vi "沿线段检测边沿点2.vi"(6 "开启线段Overlay":bool, 7 "Edge Options":T3={"Edge Polarity"=0, "Kernel Size"=5, "Width"=11, "Minimum Edge Strength"=10.0, "Interpolation Type"=enum."Bilinear Fixed", "Data Processing Method"=enum."Average"} {"Edge Polarity" items=["All Edges", "Rising Edges", "Falling Edges"]; "Minimum Edge Strength" format="%.2f"; "Width" step=2; "Kernel Size" step=2}, 8 "error in (no error)":errorcluster, 9 "终点":cluster{"X":sgl, "Y":sgl}, 10 "起点":cluster{"X":sgl, "Y":sgl}, 11 "Image":T1) -> (0 "error out":errorcluster, 2 "Edge Information":T2[](array[typedef]) {"Distance (Real-World)" format="%.2f"; "Location (Real-World)"."Y" format="%.2g"; "Location (Real-World)"."X" format="%.2f"; "Noise" format="%.2f"; "Location (Pixel)"."Y" format="%.2g"; "Location (Pixel)"."X" format="%.2f"; "Strength" format="%.2f"; "Distance (Pixel)" format="%.2f"}, 3 "Image Out":T1)   [LabVIEW 2015]
uses:
  <vilib>/vision/Measure.llb/Edge Options.ctl
  <vilib>/vision/Measure.llb/Edge Polarity.ctl
  <vilib>/vision/Measure.llb/Edge New.ctl
  <vilib>/vision/Image Controls.llb/IMAQ Image.ctl
  <vilib>/vision/NI_Vision_Development_Module.lvlib
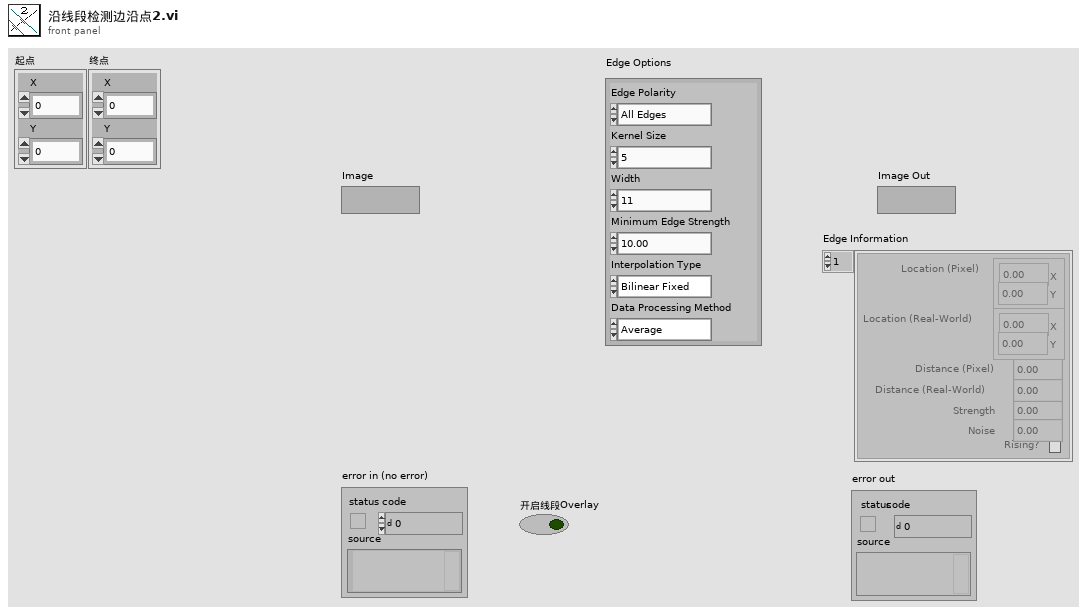
[diagram p1: front panel]
types:
  T1 = typedef "IMAQ Image.ctl" = refnum<image>
  T2 = typedef "Edge New.ctl" = cluster{"Location (Pixel)":cluster{"X":sgl, "Y":sgl}, "Location (Real-World)":cluster{"X":sgl, "Y":sgl}, "Distance (Pixel)":dbl, "Distance (Real-World)":dbl, "Strength":dbl, "Noise":dbl, "Rising?":bool}
  T3 = typedef "Edge Options.ctl" = cluster{"Edge Polarity":T4, "Kernel Size":u32, "Width":u32, "Minimum Edge Strength":sgl, "Interpolation Type":enum32{"Zero Order", "Bilinear", "Quadratic", "Cubic", "Bilinear Fixed"}, "Data Processing Method":enum32{"Average", "Median"}}
  T4 = typedef "Edge Polarity.ctl" = u32
  T5 = typedef "IMAQ Line" = cluster{"Start X":i32, "Start Y":i32, "End X":i32, "End Y":i32}
  T6 = typedef "ROI Descriptor" = cluster{"Global Rectangle":i32[], "Contours":cluster{"ID":enum32{"External", "Internal"}, "Type":u32, "Coordinates":i32[]}[]}
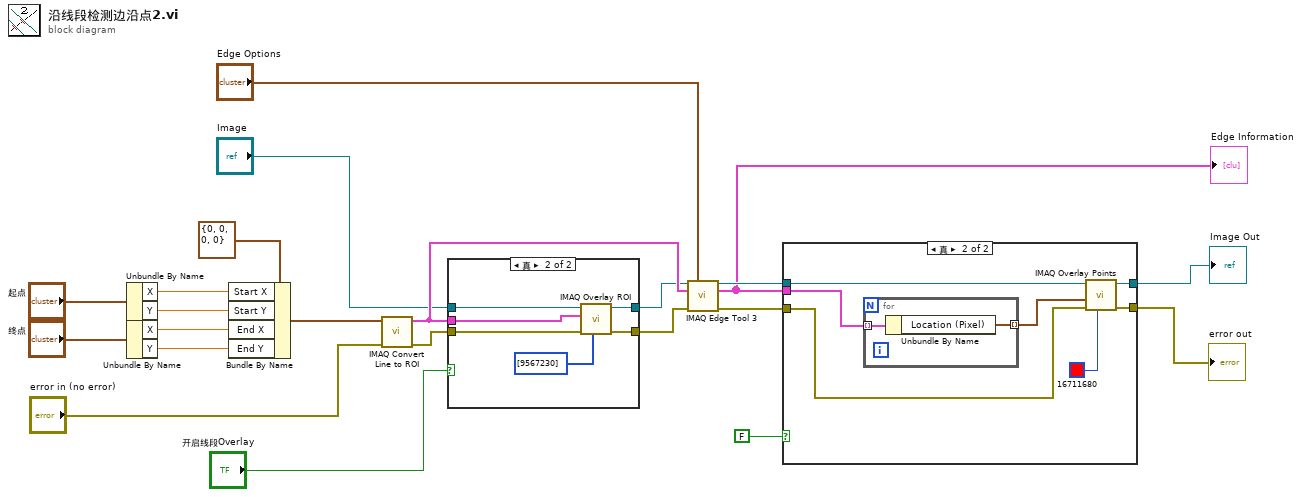
[diagram p0: block diagram]
diagram:
  n1 = Unbundle By Name("起点") -> ("X"=w6:sgl, "Y"=w5:sgl)
  n2 = Unbundle By Name("终点") -> ("X"=w3:sgl, "Y"=w2:sgl)
  n3 = Bundle By Name(cluster=T5 {"Start X"=0, "Start Y"=0, "End X"=0, "End Y"=0} ("Line"), "Start X"=w6, "Start Y"=w5, "End X"=w3, "End Y"=w2) -> (w8:T5)
  n4 = call "IMAQ Convert Line to ROI"("error in (no error)"="error in (no error)", "Line"=w8) -> ("error out"=w20:errorcluster, "ROI Descriptor"=w22:T6)  [unwired: 7 in]
  n5 = case shown="真" "开启线段Overlay" {
    tunnel: w22 -> [_ w29]
    tunnel: [w23 w28] -> w21
    tunnel: w20 -> [w24 w27]
    tunnel: [w24 w26] -> w19
    tunnel: "Image" -> [w23 w25]
    frame False {
    }
    frame True {
      n6 = call "IMAQ Overlay ROI"("Colors (Green)"=u32[] [9567230], "error in (no error)"=w27, "ROI Descriptor"=w29, "Image"=w25) -> ("error out"=w26:errorcluster, "Image Out"=w28:T1)  [unwired: 6 in]
    }
  }
  n7 = call "IMAQ Edge Tool 3"("Image"=w21, "Edge Options"="Edge Options", "ROI Descriptor"=w22, "error in (no error)"=w19) -> ("Image (duplicate)"=w17:T1, "Edge Information"=w11:T2[], "error out"=w14:errorcluster)  [unwired: 7 in, 2 out]
  "Edge Information" <- w11
  n8 = case shown="真" FALSE {
    tunnel: w17 -> [w32 w39]
    tunnel: [w31 w36] -> w15
    tunnel: w14 -> [w31 w35]
    tunnel: [w32 w34] -> w13
    tunnel: w11 -> [_ w33]
    frame False {
    }
    frame True {
      n9 = for {
        tunnel: w33 -> [w41] mode=indexing
        tunnel: [w40] -> w38 mode=indexing
        n10 = Unbundle By Name(w41) -> ("Location (Pixel)"=w40:cluster{"X":sgl, "Y":sgl})
      }
      n11 = call "IMAQ Overlay Points"("Color"=u32 16711680, "error in (no error)"=w35, "Array of Points"=w38, "Image"=w39) -> ("error out"=w36:errorcluster, "Image Out"=w34:T1)  [unwired: 6 in]
    }
  }
  "error out" <- w15
  "Image Out" <- w13
